vi "SetMirror.vi"(8 "error in (no error)":errorcluster, 9 "Front/Side":bool, 10 "Mirror":enum16{"Entrance Mirror", "Exit Mirror"}(ring), 11 "HRS_Spectrometer in":refnum<class "HRS_Spectrometer.lvclass">) -> (0 "error out":errorcluster, 3 "HRS_Spectrometer out":refnum<class "HRS_Spectrometer.lvclass">)   [LabVIEW 2023, in "HRS_Spectrometer.lvlib" / "HRS_Spectrometer.lvclass"]
uses:
  HRS_Spectrometer.lvclass
  HRS_Spectrometer.lvclass/HRS_Spectrometer.ctl
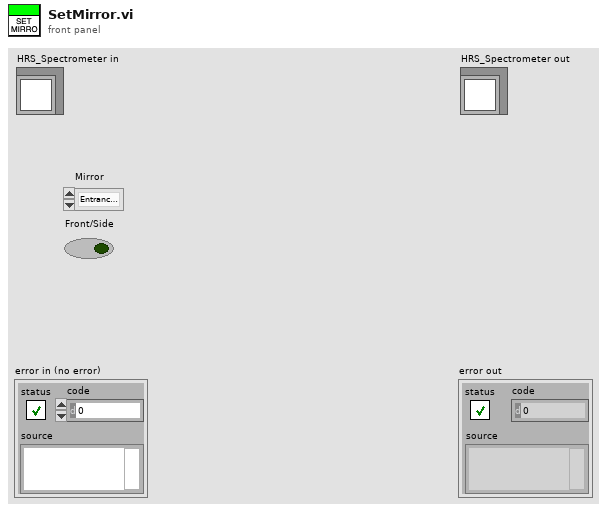
[diagram p1: front panel]
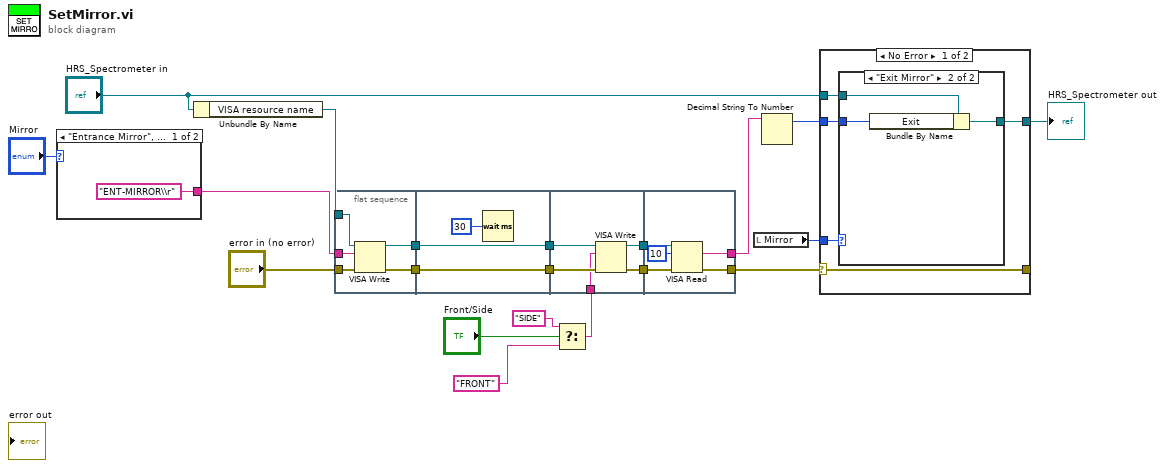
[diagram p0: block diagram]
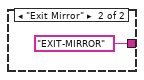
[diagram p2: hidden frame]
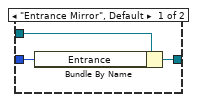
[diagram p3: hidden frame]
diagram:
  n1 = case shown="\"Entrance Mirror\", Default" "Mirror" {
    tunnel: ["ENT-MIRROR\\r" ("write buffer") "EXIT-MIRROR" ("write buffer")] -> w12
    frame "Entrance Mirror", Default {
    }
    frame "Exit Mirror" {
    }
  }
  n2 = Unbundle By Name("HRS_Spectrometer in") -> ("VISA resource name"=w13:refnum<visa-resource-name>)
  n3 = flat-sequence {
    tunnel: [w27] -> w20
    tunnel: [w26] -> w19
    tunnel: w13 -> [w25]
    tunnel: "error in (no error)" -> [w24]
    tunnel: w12 -> [w23]
    tunnel: w20 -> [w30]
    tunnel: w19 -> [w29]
    tunnel: [w30] -> w18
    tunnel: [w29] -> w17
    tunnel: w18 -> [w35]
    tunnel: [w34] -> w16
    tunnel: w17 -> [w33]
    tunnel: [w32] -> w15
    tunnel: w5 -> [w31]
    tunnel: w16 -> [w39]
    tunnel: w15 -> [w40]
    tunnel: [w38] -> w11
    tunnel: [w37] -> w14
    frame #0 {
      n4 = VISA Write(VISA resource name=w25, write buffer=w23, error in (no error)=w24) -> (VISA resource name out=w27:refnum<visa-resource-name>, error out=w26:errorcluster)  [unwired: 1 out]
    }
    frame #1 {
      n5 = Wait (ms)(milliseconds to wait=u32 30) -> ()  [unwired: 1 out]
    }
    frame #2 {
      n6 = VISA Write(VISA resource name=w35, write buffer=w31, error in (no error)=w33) -> (VISA resource name out=w34:refnum<visa-resource-name>, error out=w32:errorcluster)  [unwired: 1 out]
    }
    frame #3 {
      n7 = VISA Read(VISA resource name=w39, byte count=u32 10, error in (no error)=w40) -> (read buffer=w38:string, error out=w37:errorcluster)  [unwired: 2 out]
    }
  }
  n8 = Select(t="SIDE", s="Front/Side", f="FRONT") -> (s? t:f=w5:string)
  n9 = local read "Mirror"() -> (w1:enum16{"Entrance Mirror", "Exit Mirror"})
  n10 = Decimal String To Number(string=w11) -> (offset past number=w10:i32)  [unwired: 2 in, 1 out]
  n11 = case shown="No Error" w14 {
    selector: w14 -> [w45 w53]
    tunnel: "HRS_Spectrometer in" -> [w44 w52]
    tunnel: [w45 w53] -> _
    tunnel: [w42 w52] -> w7
    tunnel: w10 -> [w43 _]
    tunnel: w1 -> [w41 _]
    frame No Error {
      n12 = case shown="\"Exit Mirror\"" w41 {
        tunnel: w44 -> [w48 w50]
        tunnel: w43 -> [w47 w49]
        tunnel: [w46 w51] -> w42
        frame "Entrance Mirror", Default {
          n13 = Bundle By Name(cluster=w48, "Entrance"=w47) -> (w46:refnum<class "HRS_Spectrometer.lvclass">)
        }
        frame "Exit Mirror" {
          n14 = Bundle By Name(cluster=w50, "Exit"=w49) -> (w51:refnum<class "HRS_Spectrometer.lvclass">)
        }
      }
    }
    frame Error {
    }
  }
  "HRS_Spectrometer out" <- w7
